vi "DAC_set_stop-sample-count.vi"(9 "sample count":u16, 11 "FPGA VI Reference In":T1) -> (3 "FPGA VI Reference Out":T1)   [LabVIEW 2013]
uses:
  fpga-bitfile-ref.ctl
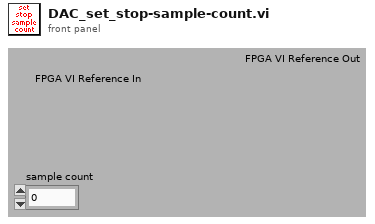
[diagram p1: front panel]
types:
  T1 = typedef "fpga-bitfile-ref.ctl" = refnum<k20>
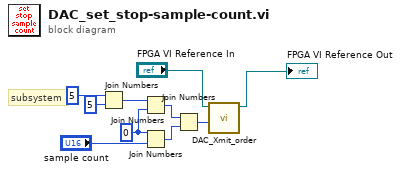
[diagram p0: block diagram]
diagram:
  w1 = u16 0 ("lo")
  # "subsystem"
  n1 = Join Numbers(hi=u8 5, lo=u8 5) -> ((hi.lo)=w7:u16)
  n2 = Join Numbers(hi=w7, lo=w1) -> ((hi.lo)=w5:u32)
  n3 = Join Numbers(hi=w1, lo="sample count") -> ((hi.lo)=w3:u32)
  n4 = Join Numbers(hi=w5, lo=w3) -> ((hi.lo)=w10:u64)
  n5 = call "DAC_Xmit_order.vi"("Order in"=w10, "FPGA VI Reference In"="FPGA VI Reference In") -> ("FPGA VI Reference Out"=→"FPGA VI Reference Out":T1)  [unwired: 9 out]
